vi "Handle REGISTERED.vi"(0 "reference":refnum<class "WAMP Client.lvclass">, 5 "error in (no error)":errorcluster, 7 "WAMP Message":T3 {"Message Codes" items=["HELLO"=1, "WELCOME"=2, "ABORT"=3, "GOODBYE"=6, "ERROR"=8, "PUBLISH"=16, "PUBLISHED"=17, "SUBSCRIBE"=32, "SUBSCRIBED"=33, "UNSUBSCRIBE"=34, "UNSUBSCRIBED"=35, "EVENT"=36, "CALL"=48, "RESULT"=59, "REGISTER"=64, "REGISTERED"=65, "UNREGISTER"=66, "UNREGISTERED"=67, "INVOCATION"=68, "YIELD"=70]}) -> (4 "reference out":refnum<class "WAMP Client.lvclass">, 6 "error out":errorcluster)   [LabVIEW 2020, in "WAMP Client.lvclass"]
uses:
  <userlib>/lvwamp/WAMP Client/WAMP Client.lvclass
  <userlib>/lvwamp/WAMP Client/TypeDef/WAMP Received Message.ctl
  <userlib>/lvwamp/WAMP Message Codes.ctl
  <userlib>/lvwamp/WAMP Client/TypeDef/Message Loop Shift Reg Data.ctl
  <userlib>/lvwamp/WAMP Client/TypeDef/REGISTER Request Data.ctl
  <userlib>/lvwamp/WAMP Client/TypeDef/REGISTERED or ERROR payload.ctl
  <userlib>/lvwamp/WAMP Client/TypeDef/WAMP Error Payload.ctl
  <userlib>/lvwamp/WAMP Client/TypeDef/INVOCATION payload.ctl
  <vilib>/JDP Science/JSONtext/JSONtext.lvlib
panel:
  out "output cluster":T1
  in  "Message Loop Shift Register Data":T1
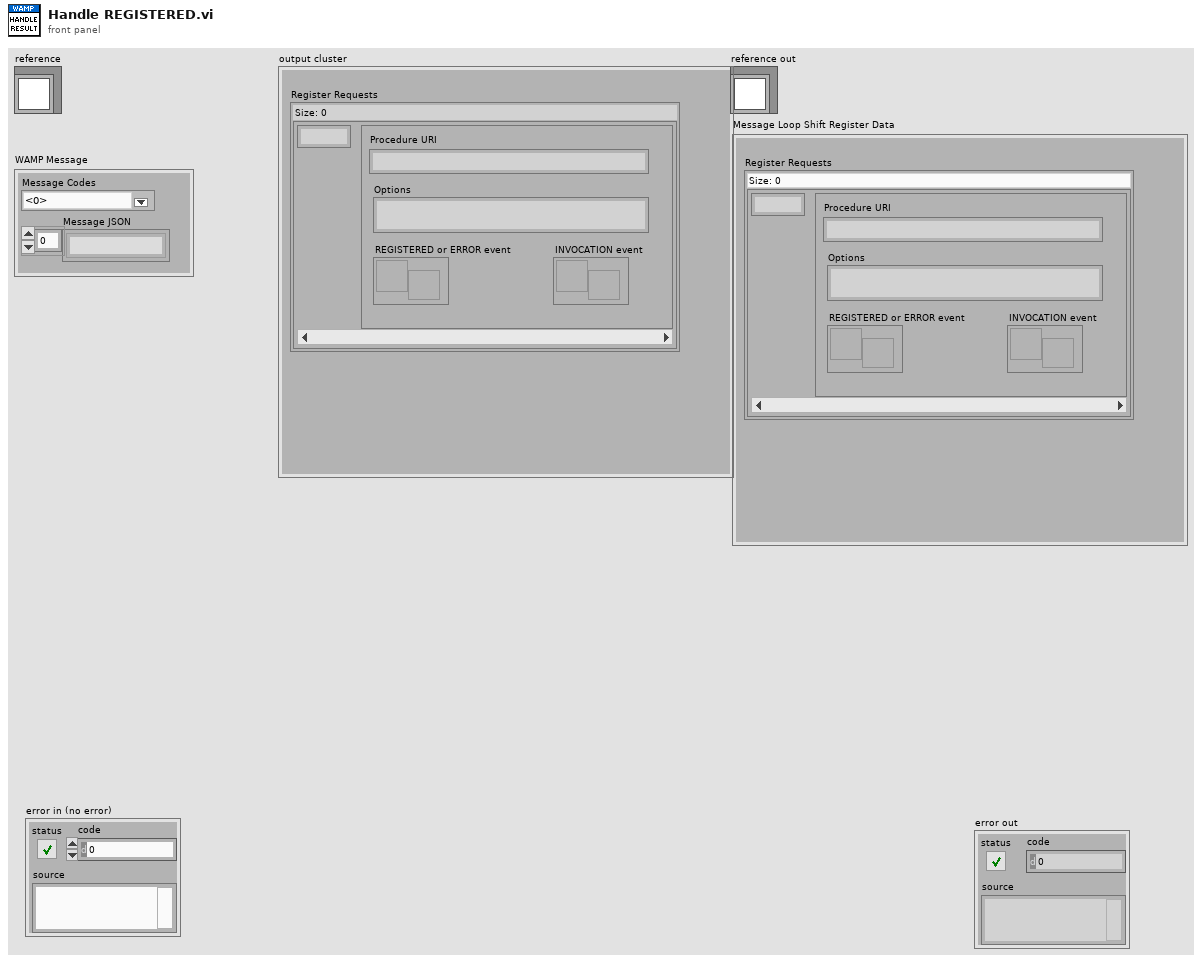
[diagram p1: front panel]
types:
  T1 = typedef "WAMP Client.lvclass/Message Loop Shift Reg Data.ctl" = cluster{"Register Requests":map{u32, T2}}
  T2 = typedef "WAMP Client.lvclass/REGISTER Request Data.ctl" = cluster{"Procedure URI":string, "Options":string, "REGISTERED or ERROR event":refnum<user-event>, "INVOCATION event":refnum<user-event>}
  T3 = typedef "WAMP Client.lvclass/WAMP Received Message.ctl" = cluster{"Message JSON":string[], "Message Codes":T4}
  T4 = typedef "WAMP Client.lvclass/WAMP Message Codes.ctl" = u16
  T5 = typedef "WAMP Client.lvclass/REGISTERED or ERROR payload.ctl" = cluster{"Register Request ID":u32, "Registration ID":u32, "Success?":bool, "Cluster":T6, "Procedure URI":string}
  T6 = typedef "WAMP Client.lvclass/WAMP Error Payload.ctl" = cluster{"Arguments Payload":string[], "ArgumentKw Payload":string, "Error URI":string, "Error?":bool}
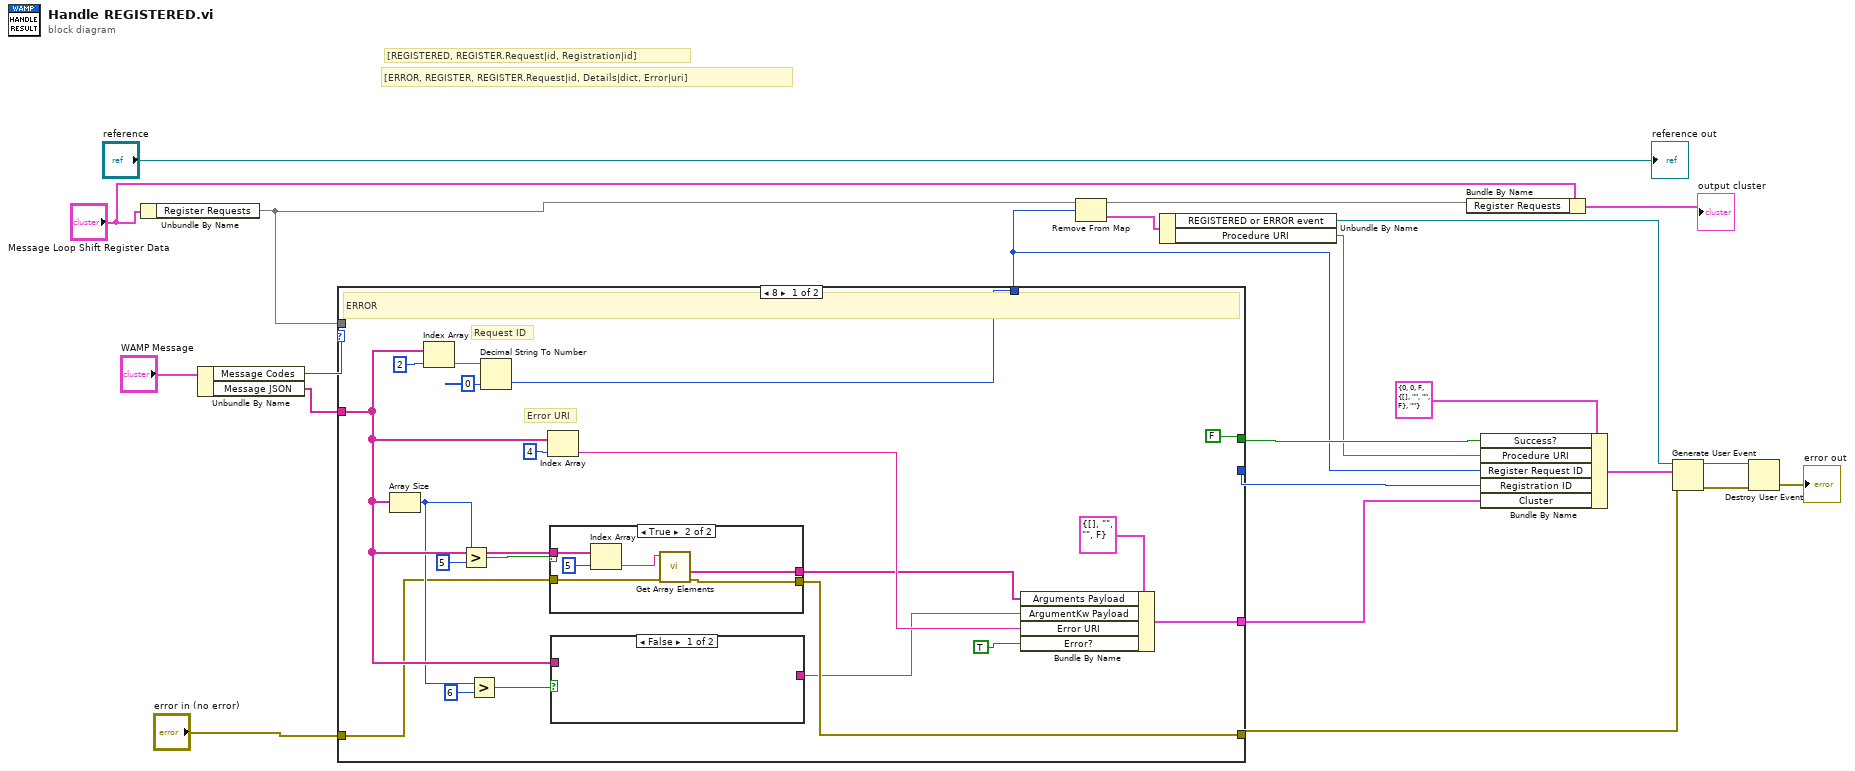
[diagram p0: block diagram]
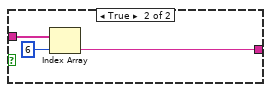
[diagram p2: hidden frame]
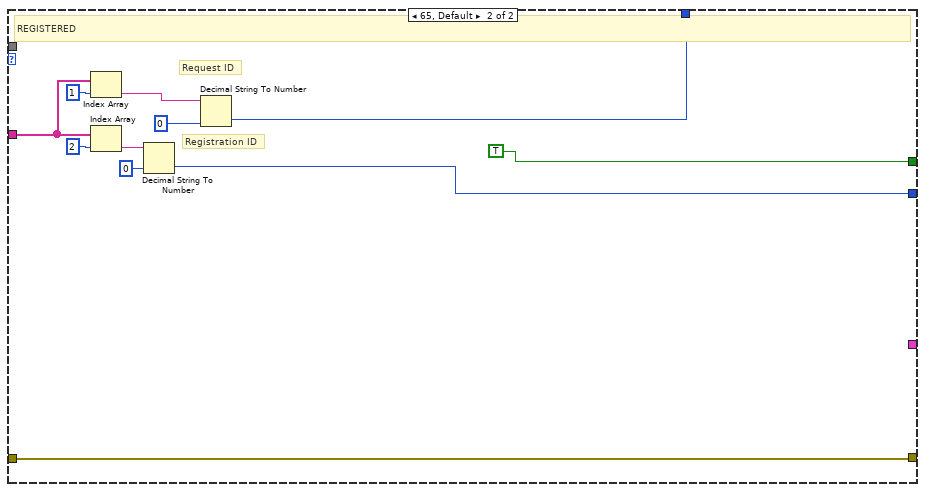
[diagram p4: hidden frame]
diagram:
  # "[ERROR, REGISTER, REGISTER.Request|id, Details|dict, Error|uri]"
  # "[REGISTERED, REGISTER.Request|id, Registration|id]"
  n1 = Unbundle By Name("Message Loop Shift Register Data") -> ("Register Requests"=w10:map{u32, T2})
  n2 = Unbundle By Name("WAMP Message") -> ("Message Codes"=w18:T4, "Message JSON"=w17:string[])
  n3 = case shown="8" w18 {
    tunnel: w17 -> [w35 w56]
    tunnel: [w38 w55] -> w8
    tunnel: "error in (no error)" -> [w31 w53]
    tunnel: [w30 w53] -> w20
    tunnel: [FALSE ("Success?") TRUE ("Success?")] -> w21
    tunnel: w10 -> [_ _]
    tunnel: [_ w54] -> w7
    tunnel: [w23 _] -> w6
    frame 8 {
      # "Request ID"
      # "Error URI"
      # "ERROR"
      n4 = Array Size(array=w35) -> (size(s)=w32:i32)
      n5 = Index Array(array=w35, index=u32 2) -> (element=w41:string)
      n6 = Greater?(x=w32, y=5) -> (0:w36:bool)
      n7 = Greater?(x=w32, y=6) -> (0:w33:bool)
      n8 = Decimal String To Number(string=w41, default (0L)=u32 0) -> (number=w38:u32)  [unwired: 1 in, 1 out]
      n9 = Index Array(array=w35, index=4) -> (element=w27:string)
      n10 = case shown="True" w36 {
        tunnel: w35 -> [_ w51]
        tunnel: [_ w50] -> w26
        tunnel: w31 -> [w46 w48]
        tunnel: [w46 w47] -> w30
        frame False {
        }
        frame True {
          n11 = Index Array(array=w51, index=5) -> (element=w49:string)
          n12 = call <vilib>:"Get Array Elements.vi"("error in (no error)"=w48, "JSON"=w49) -> ("error out"=w47:errorcluster, "<JSON>"=w50:string[])  [unwired: 7 in, 1 out]
        }
      }
      n13 = case shown="False" w33 {
        tunnel: [_ w44] -> w25
        tunnel: w35 -> [_ w43]
        frame False {
        }
        frame True {
          n14 = Index Array(array=w43, index=6) -> (element=w44:string)
        }
      }
      n15 = Bundle By Name(cluster=T6 {"Arguments Payload"=[], "ArgumentKw Payload"="", "Error URI"="", "Error?"=FALSE} ("Cluster"), "Arguments Payload"=w26, "ArgumentKw Payload"=w25, "Error URI"=w27, "Error?"=TRUE ("status")) -> (w23:T6)
    }
    frame 65, Default {
      # "Request ID"
      # "Registration ID"
      # "REGISTERED"
      n16 = Index Array(array=w56, index=1) -> (element=w59:string)
      n17 = Index Array(array=w56, index=2) -> (element=w62:string)
      n18 = Decimal String To Number(string=w62, default (0L)=u32 0) -> (number=w54:u32)  [unwired: 1 in, 1 out]
      n19 = Decimal String To Number(string=w59, default (0L)=u32 0) -> (number=w55:u32)  [unwired: 1 in, 1 out]
    }
  }
  n20 = Remove From Map(10:w8, 11:w10) -> (1:w16:T2, 3:w4:map{u32, T2})  [unwired: 1 out]
  n21 = Unbundle By Name(w16) -> ("REGISTERED or ERROR event"=w13:refnum<user-event>, "Procedure URI"=w1:string)
  n22 = Bundle By Name(cluster="Message Loop Shift Register Data", "Register Requests"=w4) -> (→"output cluster":T1)
  n23 = Bundle By Name(cluster=T5 {"Register Request ID"=0, "Registration ID"=0, "Success?"=FALSE, "Cluster"={"Arguments Payload"=[], "ArgumentKw Payload"="", "Error URI"="", "Error?"=FALSE}, "Procedure URI"=""} ("REGISTERED or ERROR payload"), "Success?"=w21, "Procedure URI"=w1, "Register Request ID"=w8, "Registration ID"=w7, "Cluster"=w6) -> (w11:T5)
  n24 = Generate User Event(user event=w13, event data cluster=w11, error in=w20) -> (user event out=w14:refnum<user-event>, error out=w15:errorcluster)  [unwired: 1 in]
  n25 = Destroy User Event(user event=w14, error in=w15) -> (error out=→"error out":errorcluster)
  "reference out" <- "reference"
